vi "Clear.vi"(8 "error in (no error)":errorcluster, 11 "dataClass in":refnum<class "SR430Class.lvclass">) -> (0 "error out":errorcluster, 3 "dataClass out":refnum<class "SR430Class.lvclass">)   [LabVIEW 2015, in "SR430Class.lvclass"]
uses:
  class/SR430Class.lvclass
  class/SR430Class.lvclass/SR430Class.ctl
  support/SR430 Driver/SR430Driver.lvlib
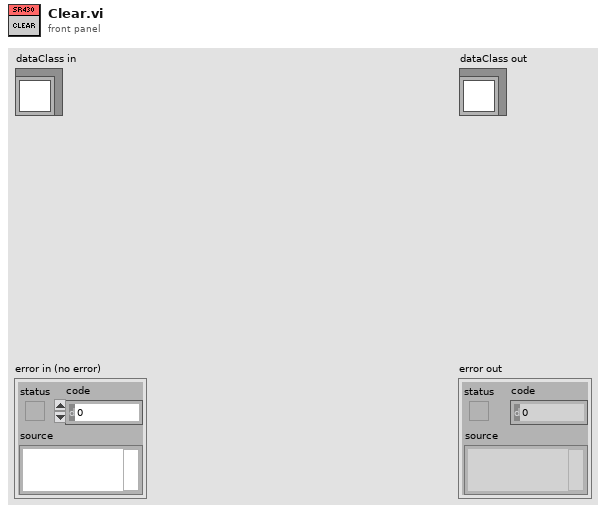
[diagram p1: front panel]
types:
  T1 = typedef "SR430Driver.lvlib/SR430_VISA Control.ctl" = cluster{"VISA resource name":refnum<visa-resource-name>}
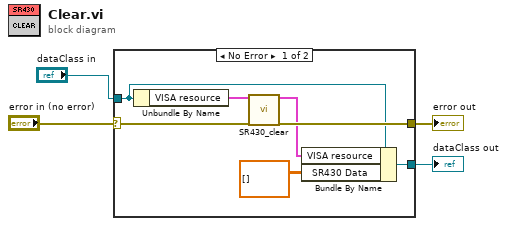
[diagram p0: block diagram]
diagram:
  n1 = case shown="No Error" "error in (no error)" {
    selector: "error in (no error)" -> [w10 w13]
    tunnel: [w9 w13] -> w3
    tunnel: [w6 w12] -> w1
    tunnel: "dataClass in" -> [w8 w12]
    frame No Error {
      n2 = Unbundle By Name(w8) -> ("VISA resource"=w11:T1)
      n3 = call "SR430_clear.vi"("address"=w11, "error in (no error)"=w10) -> ("address out"=w7:T1, "error out"=w9:errorcluster)  [unwired: 16 in]
      n4 = Bundle By Name(cluster=w8, "VISA resource"=w7, "SR430 Data"=dbl[][] []) -> (w6:refnum<class "SR430Class.lvclass">)
    }
    frame Error {
    }
  }
  "error out" <- w3
  "dataClass out" <- w1
